vi "测试类型1自动测试一组.vi"() -> ()   [LabVIEW 2010]
uses:
  全局量/试验配置信息.vi
panel:
  in  "测试值":dbl[](array[numeric])
  out "EVENT_KEY":string
  out "bRece":bool
  out "bSend":bool
  out "第几个":i32
  out "bStop":bool
  out "数据组数":i32
  out "第几组":i32
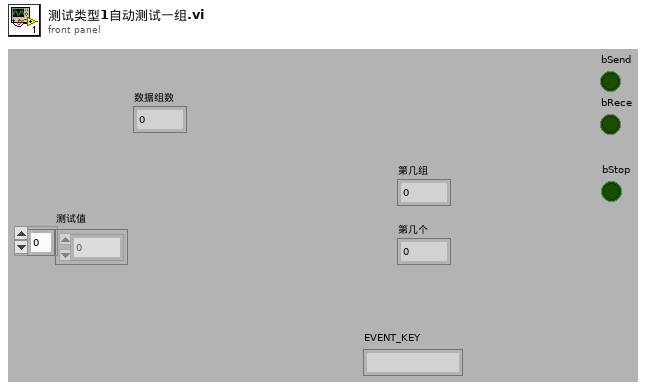
[diagram p1: front panel]
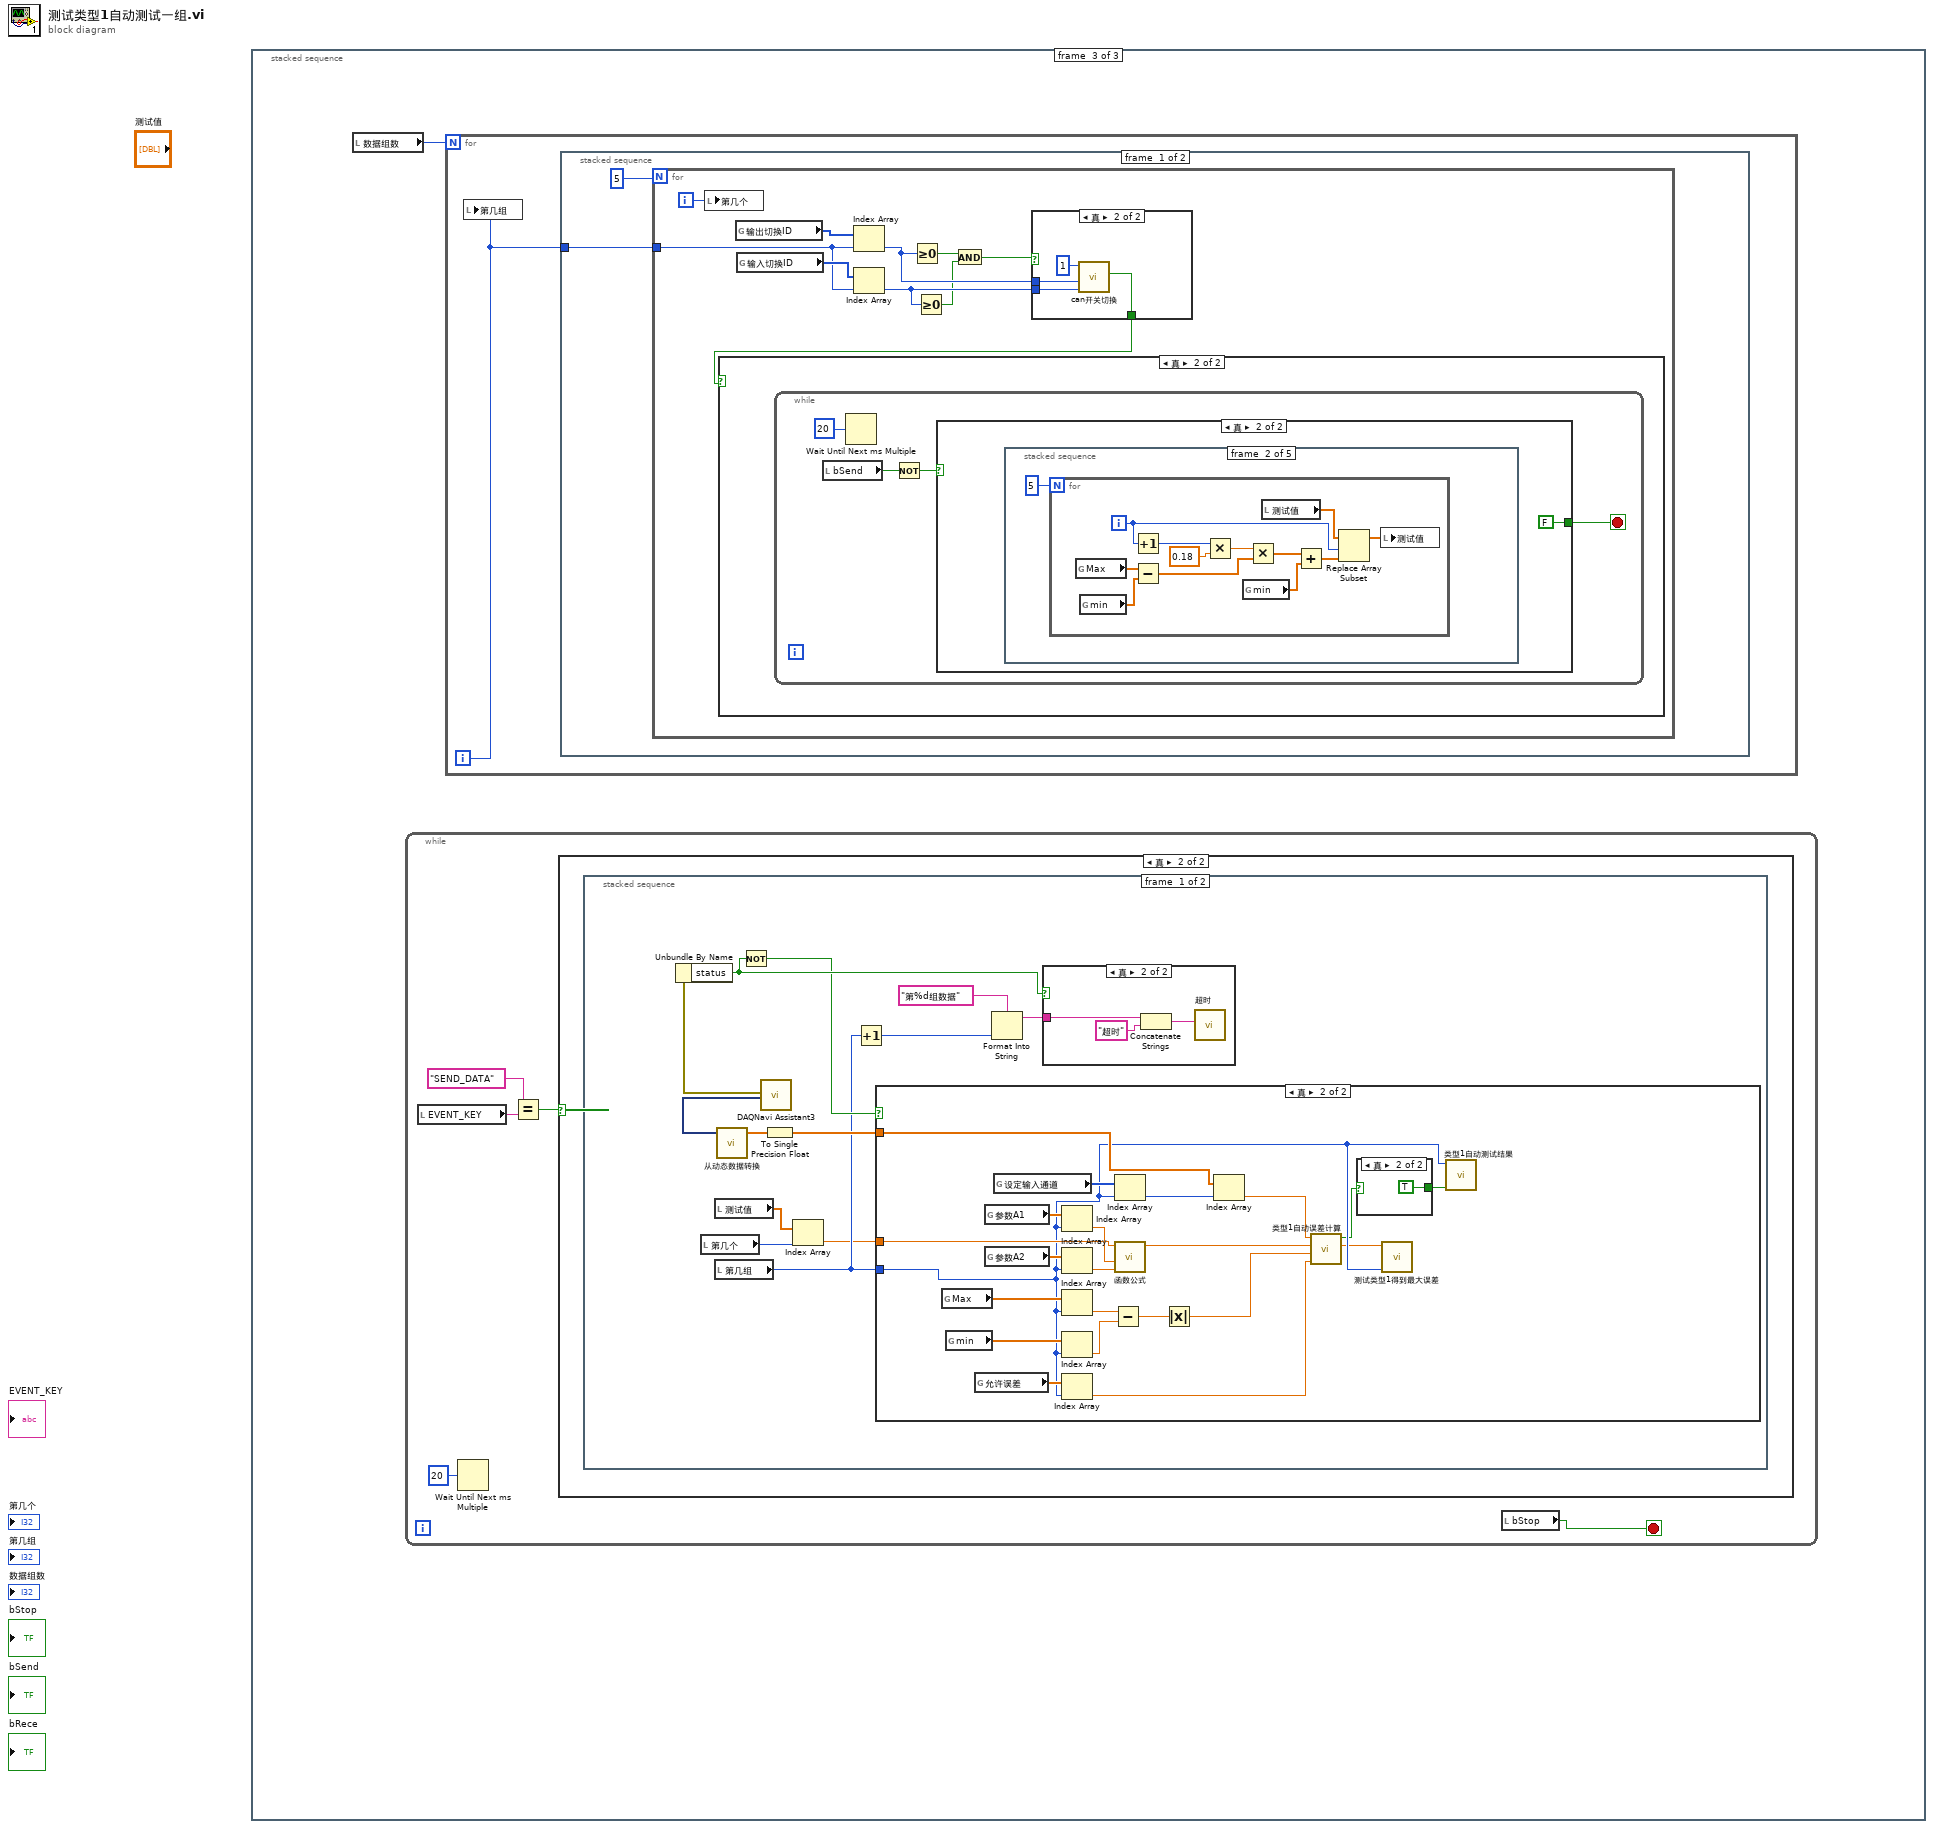
[diagram p0: block diagram]
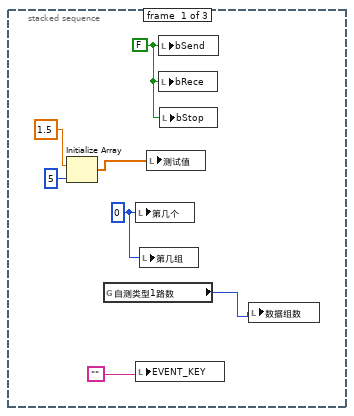
[diagram p2: hidden frame]
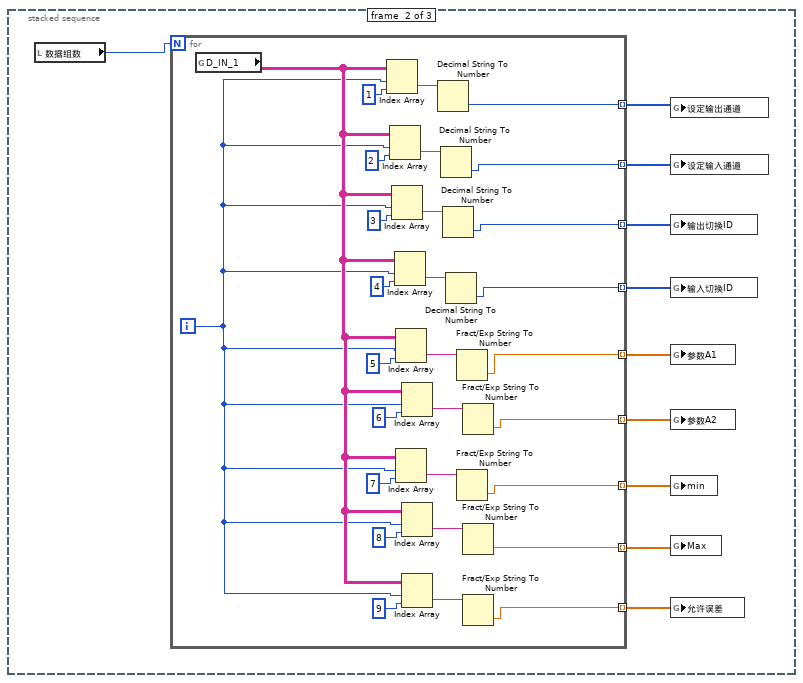
[diagram p3: hidden frame]
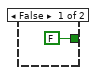
[diagram p7: hidden frame]
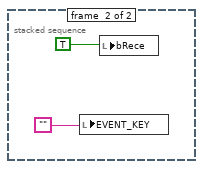
[diagram p8: hidden frame]
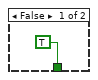
[diagram p9: hidden frame]
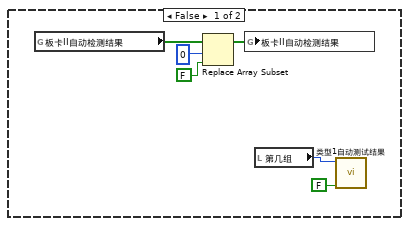
[diagram p10: hidden frame]
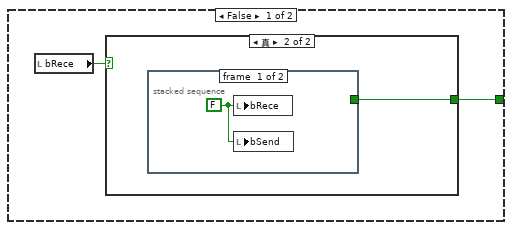
[diagram p11: hidden frame]
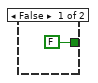
[diagram p12: hidden frame]
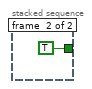
[diagram p13: hidden frame]
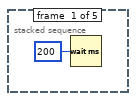
[diagram p14: hidden frame]
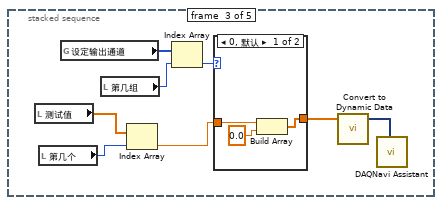
[diagram p15: hidden frame]
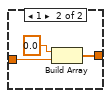
[diagram p16: hidden frame]
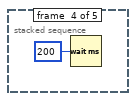
[diagram p17: hidden frame]
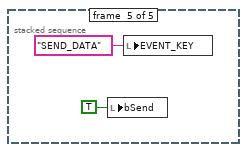
[diagram p18: hidden frame]
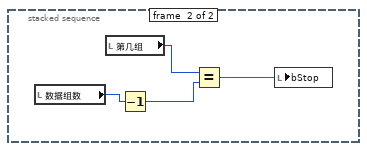
[diagram p19: hidden frame]
diagram:
  n1 = stacked-sequence {
    frame #0 {
      w6 = FALSE
      w7 = 0 ("同步A")
      n2 = Initialize Array(1.5 ("数值"), 5 ("维数大小")) -> (w2:dbl[])
      n3 = global read "试验配置信息.vi" "自测类型1路数"() -> (w1:i32)
      n4 = local write "第几个"(w7) -> ()
      n5 = local write "EVENT_KEY"("") -> ()
      n6 = local write "第几组"(w7) -> ()
      n7 = local write "测试值"(w2) -> ()
      n8 = local write "bSend"(w6) -> ()
      n9 = local write "bRece"(w6) -> ()
      n10 = local write "bStop"(w6) -> ()
      n11 = local write "数据组数"(w1) -> ()
    }
    frame #1 {
      n12 = local read "数据组数"() -> (w8:i32)
      n13 = for {
        N: w8 -> [_]
        tunnel: [w26] -> w9 mode=indexing
        tunnel: [w25] -> w10 mode=indexing
        tunnel: [w24] -> w11 mode=indexing
        tunnel: [w23] -> w12 mode=indexing
        tunnel: [w22] -> w13 mode=indexing
        tunnel: [w21] -> w14 mode=indexing
        tunnel: [w20] -> w15 mode=indexing
        tunnel: [w19] -> w16 mode=indexing
        tunnel: [w18] -> w17 mode=indexing
        i -> [w27]
        n14 = global read "试验配置信息.vi" "D_IN_1"() -> (w28:string[][])
        n15 = Index Array(array=w28, index (row)=w27, index (col)=1 ("禁用的索引 (列)")) -> (element=w46:string)
        n16 = Index Array(array=w28, index (row)=w27, index (col)=2 ("禁用的索引 (列)")) -> (element=w43:string)
        n17 = Index Array(array=w28, index (row)=w27, index (col)=3 ("禁用的索引 (列)")) -> (element=w39:string)
        n18 = Index Array(array=w28, index (row)=w27, index (col)=4 ("禁用的索引 (列)")) -> (element=w42:string)
        n19 = Index Array(array=w28, index (row)=w27, index (col)=5 ("禁用的索引 (列)")) -> (element=w37:string)
        n20 = Index Array(array=w28, index (row)=w27, index (col)=7 ("禁用的索引 (列)")) -> (element=w32:string)
        n21 = Index Array(array=w28, index (row)=w27, index (col)=6 ("禁用的索引 (列)")) -> (element=w36:string)
        n22 = Index Array(array=w28, index (row)=w27, index (col)=8 ("禁用的索引 (列)")) -> (element=w33:string)
        n23 = Index Array(array=w28, index (row)=w27, index (col)=9 ("禁用的索引 (列)")) -> (element=w30:string)
        n24 = Decimal String To Number(string=w46) -> (number=w26:i32)  [unwired: 2 in, 1 out]
        n25 = Decimal String To Number(string=w43) -> (number=w25:i32)  [unwired: 2 in, 1 out]
        n26 = Decimal String To Number(string=w39) -> (number=w24:i32)  [unwired: 2 in, 1 out]
        n27 = Decimal String To Number(string=w42) -> (number=w23:i32)  [unwired: 2 in, 1 out]
        n28 = Fract/Exp String To Number(string=w37) -> (number=w22:dbl)  [unwired: 3 in, 1 out]
        n29 = Fract/Exp String To Number(string=w32) -> (number=w20:dbl)  [unwired: 3 in, 1 out]
        n30 = Fract/Exp String To Number(string=w36) -> (number=w21:dbl)  [unwired: 3 in, 1 out]
        n31 = Fract/Exp String To Number(string=w33) -> (number=w19:dbl)  [unwired: 3 in, 1 out]
        n32 = Fract/Exp String To Number(string=w30) -> (number=w18:dbl)  [unwired: 3 in, 1 out]
      }
      n33 = global write "试验配置信息.vi" "设定输出通道"(w9) -> ()
      n34 = global write "试验配置信息.vi" "设定输入通道"(w10) -> ()
      n35 = global write "试验配置信息.vi" "输出切换ID"(w11) -> ()
      n36 = global write "试验配置信息.vi" "输入切换ID"(w12) -> ()
      n37 = global write "试验配置信息.vi" "参数A1"(w13) -> ()
      n38 = global write "试验配置信息.vi" "参数A2"(w14) -> ()
      n39 = global write "试验配置信息.vi" "min"(w15) -> ()
      n40 = global write "试验配置信息.vi" "Max"(w16) -> ()
      n41 = global write "试验配置信息.vi" "允许误差"(w17) -> ()
    }
    frame #2 {
      n42 = local read "数据组数"() -> (w47:i32)
      n43 = while {
        stop <- w48 stop-if-true
        n44 = local read "EVENT_KEY"() -> (w51:string)
        n45 = Wait Until Next ms Multiple(millisecond multiple=u32 20 ("毫秒倍数")) -> ()  [unwired: 1 out]
        n46 = Equal?(x="SEND_DATA" ("EVENT_KEY"), y=w51) -> (x = y?=w50:bool)
        n47 = case shown="真" w50 {
          frame False {
          }
          frame True {
            n48 = stacked-sequence {
              frame #0 {
                n49 = local read "第几个"() -> (w54:i32)
                n50 = local read "测试值"() -> (w55:dbl[])
                n51 = local read "第几组"() -> (w56:i32)
                n52 = call "DAQNavi Assistant3"() -> ("error out"=w61:errorcluster, "data out(DDT)"=w62:dynamicdata)  [unwired: 2 in, 16 out]
                n53 = Unbundle By Name(w61) -> ("status"=w65:bool)
                n54 = call "从动态数据转换"("Dynamic Data Type"=w62) -> ("Array"=w63:dbl[])  [unwired: 3 in]
                n55 = Not(x=w65) -> (.not. x?=w60:bool)
                n56 = To Single Precision Float(number=w63) -> (single precision float=w64:sgl[])
                n57 = Index Array(array=w55, index=w54) -> (element=w53:dbl)
                n58 = Increment(x=w56) -> (x+1=w59:i32)
                n59 = case shown="真" w60 {
                  tunnel: w64 -> [_ w88]
                  tunnel: w56 -> [_ w75]
                  tunnel: w53 -> [_ w76]
                  frame False {
                  }
                  frame True {
                    n60 = global read "试验配置信息.vi" "Max"() -> (w84:dbl[])
                    n61 = global read "试验配置信息.vi" "min"() -> (w85:dbl[])
                    n62 = global read "试验配置信息.vi" "允许误差"() -> (w83:dbl[])
                    n63 = global read "试验配置信息.vi" "参数A1"() -> (w87:dbl[])
                    n64 = global read "试验配置信息.vi" "参数A2"() -> (w86:dbl[])
                    n65 = global read "试验配置信息.vi" "设定输入通道"() -> (w90:u32[])
                    n66 = Index Array(array=w87, index=w75) -> (element=w77:dbl)
                    n67 = Index Array(array=w86, index=w75) -> (element=w79:dbl)
                    n68 = Index Array(array=w84, index=w75) -> (element=w81:dbl)
                    n69 = Index Array(array=w85, index=w75) -> (element=w80:dbl)
                    n70 = Index Array(array=w83, index=w75) -> (element=w71:dbl)
                    n71 = Subtract(x=w81, y=w80) -> (x-y=w82:dbl)
                    n72 = Index Array(array=w90, index=w75) -> (element=w89:u32)
                    n73 = call "函数公式.vi"("参数 b"=w79, "参数 a"=w77, "设定值 1"=w76) -> ("y"=w73:dbl)  [unwired: 5 in, 1 out]
                    n74 = Absolute Value(x=w82) -> (abs(x)=w72:dbl)
                    n75 = Index Array(array=w88, index=w89) -> (element=w74:sgl)
                    n76 = call "类型1自动误差计算.vi"("允许误差"=w71, "模拟量量程范围"=w72, "设定值_1"=w73, "反馈值_1"=w74) -> ("误差_1"=w70:dbl, "合格_1?"=w69:bool)  [unwired: 5 in, 1 out]
                    n77 = case shown="真" w69 {
                      tunnel: [FALSE TRUE] -> w78
                      frame False {
                      }
                      frame True {
                      }
                    }
                    n78 = call "测试类型1得到最大误差.vi"("第几组"=w75, "新误差值"=w70) -> ()  [unwired: 10 in]
                    n79 = call "类型1自动测试结果.vi"("合格?"=w78, "第几组"=w75) -> ()  [unwired: 10 in]
                  }
                }
                n80 = Format Into String(format string="第%d组数据" ("格式字符串"), w59) -> (resulting string=w58:string)  [unwired: 2 in, 1 out]
                n81 = case shown="真" w65 {
                  tunnel: w58 -> [_ w68]
                  frame False {
                  }
                  frame True {
                    n82 = Concatenate Strings(w68, "超时" ("格式字符串")) -> (w66:string)
                    n83 = call "超时"("Message"=w66) -> ()  [unwired: 9 in, 2 out]
                  }
                }
              }
              frame #1 {
                n84 = local write "EVENT_KEY"("") -> ()
                n85 = local write "bRece"(TRUE) -> ()
              }
            }
          }
        }
        n86 = local read "bStop"() -> (w48:bool)
      }
      n87 = for {
        N: w47 -> [_]
        i -> [w95]
        n88 = local write "第几组"(w95) -> ()
        n89 = stacked-sequence {
          tunnel: w95 -> [w96 _]
          frame #0 {
            n90 = for {
              N: 5 -> [_]
              tunnel: w96 -> [w104]
              i -> [w107]
              n91 = local write "第几个"(w107) -> ()
              n92 = global read "试验配置信息.vi" "输出切换ID"() -> (w106:i32[])
              n93 = global read "试验配置信息.vi" "输入切换ID"() -> (w105:i32[])
              n94 = Index Array(array=w106, index=w104) -> (element=w103:i32)
              n95 = Index Array(array=w105, index=w104) -> (element=w102:i32)
              n96 = Greater Or Equal To 0?(x=w103) -> (x >= 0?=w101:bool)
              n97 = Greater Or Equal To 0?(x=w102) -> (x >= 0?=w100:bool)
              n98 = And(x=w101, y=w100) -> (x .and. y?=w99:bool)
              n99 = case shown="真" w99 {
                tunnel: w103 -> [_ w111]
                tunnel: w102 -> [_ w110]
                tunnel: [TRUE w109] -> w98
                frame False {
                }
                frame True {
                  n100 = call "can开关切换.vi"("输入切换ID"=w110, "输出切换ID"=w111, "函数类型"=1) -> ("成功？"=w109:bool)  [unwired: 7 in]
                }
              }
              n101 = case shown="真" w98 {
                frame False {
                  n102 = global read "试验配置信息.vi" "板卡II自动检测结果"() -> (w118:bool[])
                  n103 = Replace Array Subset(array=w118, new element=FALSE, index=0 ("索引")) -> (w117:bool[])
                  n104 = global write "试验配置信息.vi" "板卡II自动检测结果"(w117) -> ()
                  n105 = local read "第几组"() -> (w113:i32)
                  n106 = call "类型1自动测试结果.vi"("合格?"=FALSE, "第几组"=w113) -> ()  [unwired: 10 in]
                }
                frame True {
                  n107 = while {
                    stop <- w120 stop-if-true
                    n108 = local read "bSend"() -> (w122:bool)
                    n109 = Wait Until Next ms Multiple(millisecond multiple=u32 20 ("毫秒倍数")) -> ()  [unwired: 1 out]
                    n110 = Not(x=w122) -> (.not. x?=w121:bool)
                    n111 = case shown="真" w121 {
                      tunnel: [w123 FALSE] -> w120
                      frame False {
                        n112 = local read "bRece"() -> (w124:bool)
                        n113 = case shown="真" w124 {
                          tunnel: [FALSE w126] -> w123
                          frame False {
                          }
                          frame True {
                            n114 = stacked-sequence {
                              tunnel: [_ TRUE] -> w126
                              frame #0 {
                                w127 = FALSE
                                n115 = local write "bRece"(w127) -> ()
                                n116 = local write "bSend"(w127) -> ()
                              }
                              frame #1 {
                              }
                            }
                          }
                        }
                      }
                      frame True {
                        n117 = stacked-sequence {
                          frame #0 {
                            n118 = Wait (ms)(milliseconds to wait=u32 200 ("等待时间（毫秒）")) -> ()  [unwired: 1 out]
                          }
                          frame #1 {
                            n119 = for {
                              N: 5 -> [_]
                              i -> [w135]
                              n120 = global read "试验配置信息.vi" "Max"() -> (w143:dbl[])
                              n121 = global read "试验配置信息.vi" "min"() -> (w142:dbl[])
                              n122 = Increment(x=w135) -> (x+1=w141:i32)
                              n123 = Subtract(x=w143, y=w142) -> (x-y=w138:dbl[])
                              n124 = Multiply(x=w141, y=0.18) -> (x*y=w139:dbl)
                              n125 = global read "试验配置信息.vi" "min"() -> (w134:dbl[])
                              n126 = Multiply(x=w139, y=w138) -> (x*y=w133:dbl[])
                              n127 = local read "测试值"() -> (w137:dbl[])
                              n128 = Add(x=w133, y=w134) -> (x+y=w132:dbl[])
                              n129 = Replace Array Subset(array=w137, new element=w132, index=w135) -> (w136:dbl[])
                              n130 = local write "测试值"(w136) -> ()
                            }
                          }
                          frame #2 {
                            n131 = local read "测试值"() -> (w146:dbl[])
                            n132 = local read "第几个"() -> (w144:i32)
                            n133 = global read "试验配置信息.vi" "设定输出通道"() -> (w148:u32[])
                            n134 = local read "第几组"() -> (w151:i32)
                            n135 = Index Array(array=w146, index=w144) -> (element=w145:dbl)
                            n136 = Index Array(array=w148, index=w151) -> (element=w149:u32)
                            n137 = case shown="0, 默认" w149 {
                              tunnel: [w154 w157] -> w150
                              tunnel: w145 -> [w152 w155]
                              frame 0, Default {
                                n138 = Build Array(w152, 0.0) -> (w154:dbl[])
                              }
                              frame 1 {
                                n139 = Build Array(0.0, w155) -> (w157:dbl[])
                              }
                            }
                            n140 = call "Convert to Dynamic Data"("Array"=w150) -> ("Dynamic Data Type"=w147:dynamicdata)  [unwired: 3 out]
                            n141 = call "DAQNavi Assistant"("data in(DDT)"=w147) -> ()  [unwired: 2 in, 17 out]
                          }
                          frame #3 {
                            n142 = Wait (ms)(milliseconds to wait=u32 200 ("等待时间（毫秒）")) -> ()  [unwired: 1 out]
                          }
                          frame #4 {
                            n143 = local write "bSend"(TRUE) -> ()
                            n144 = local write "EVENT_KEY"("SEND_DATA" ("EVENT_KEY")) -> ()
                          }
                        }
                      }
                    }
                  }
                }
              }
            }
          }
          frame #1 {
            n145 = local read "数据组数"() -> (w162:i32)
            n146 = local read "第几组"() -> (w164:i32)
            n147 = Decrement(x=w162) -> (x-1=w161:i32)
            n148 = Equal?(x=w164, y=w161) -> (x = y?=w163:bool)
            n149 = local write "bStop"(w163) -> ()
          }
        }
      }
    }
  }
